vi "ERIO RT Send Notification Messages.vi"(8 "error in (no error)":errorcluster, 9 "AWS Variables In":T1, 10 "Message Body":string, 11 "Supervisory Variables In":T2={"Alarm Threshold"=0.0, "Shutdown"=FALSE, "Enable SNS Alarm"=FALSE, "Enable SNS Stage Notification"=FALSE, "Enable SQS Notification"=FALSE, "Enable S3 TDMS Signal Capture"=FALSE, "Enable SystemLink Signal Capture"=FALSE, "Capture Signal"=FALSE, "Server Update"=FALSE, "AWS Access Key"="", "AWS Secret Key"="", "Phone Number"="", "Region"=enum."us-east-1", "AWS SQS Queue"="mynicloud-demotest2", "AWS S3 Bucket"="mynicloud-demotest2"}) -> (0 "error out":errorcluster, 1 "AWS Variables Out":T1)   [LabVIEW 2017]
doc: "Send out relevant notification messages.\n\nJames Tillett PE\nEndeavor Engineering Inc.\nwww.endeavoreng.com"
uses:
  Controls/ERIO Supervisory Variables.ctl
  <vilib>/AWS Toolkit/Core/HTTP Request/Region.ctl
  Controls/ERIO AWS Toolkit Variables.ctl
  <vilib>/AWS Toolkit/SQS/Queue/Queue.lvclass
  <vilib>/AWS Toolkit/SNS/Phone Number/Phone Number.lvclass
  <vilib>/AWS Toolkit/S3/Bucket/Bucket.lvclass
  <vilib>/AWS Toolkit/Core/HTTP Request/HTTP Request.lvclass
panel:
  out "Supervisory Variables oUT":T2={"Alarm Threshold"=0.0, "Shutdown"=FALSE, "Enable SNS Alarm"=FALSE, "Enable SNS Stage Notification"=FALSE, "Enable SQS Notification"=FALSE, "Enable S3 TDMS Signal Capture"=FALSE, "Enable SystemLink Signal Capture"=FALSE, "Capture Signal"=FALSE, "Server Update"=FALSE, "AWS Access Key"="", "AWS Secret Key"="", "Phone Number"="", "Region"=enum."us-east-1", "AWS SQS Queue"="mynicloud-demotest2", "AWS S3 Bucket"="mynicloud-demotest2"}
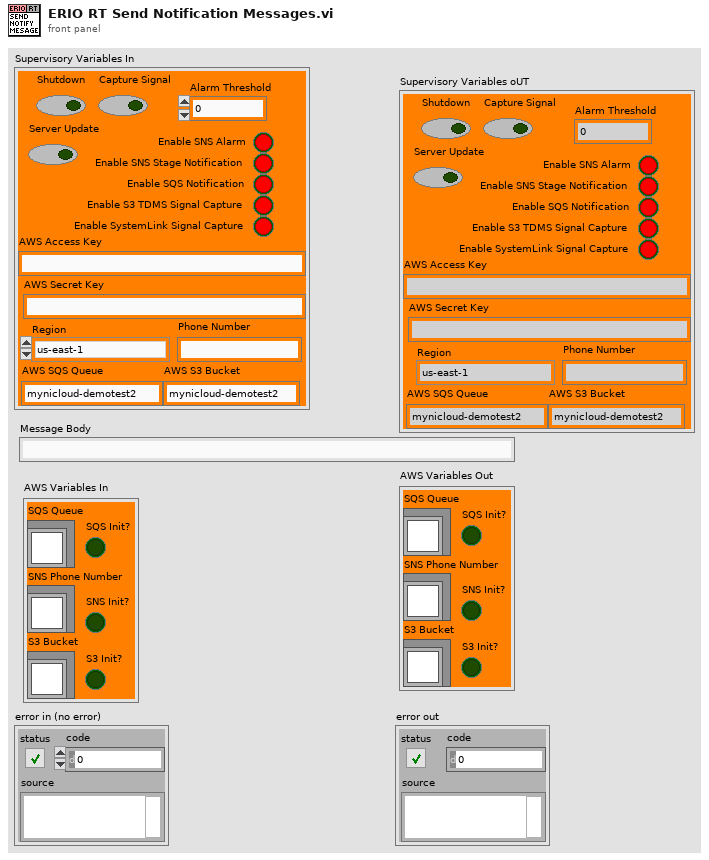
[diagram p1: front panel]
types:
  T1 = typedef "ERIO AWS Toolkit Variables.ctl" = cluster{"SQS Queue":refnum<class "Queue.lvclass">, "SNS Phone Number":refnum<class "Phone Number.lvclass">, "S3 Bucket":refnum<class "Bucket.lvclass">, "SQS Init?":bool, "S3 Init?":bool, "SNS Init?":bool}
  T2 = typedef "ERIO Supervisory Variables.ctl" = cluster{"Alarm Threshold":dbl, "Shutdown":bool, "Enable SNS Alarm":bool, "Enable SNS Stage Notification":bool, "Enable SQS Notification":bool, "Enable S3 TDMS Signal Capture":bool, "Enable SystemLink Signal Capture":bool, "Capture Signal":bool, "Server Update":bool, "AWS Access Key":string, "AWS Secret Key":string, "Phone Number":string, "Region":T3, "AWS SQS Queue":string, "AWS S3 Bucket":string}
  T3 = typedef "NI_AWS_Core.lvlib/HTTP Request.lvclass/Region.ctl" = enum16{"us-east-1", "us-east-2", "us-west-1", "us-west-2", "ap-northeast-1", "ap-northeast-2", "ap-southeast-1", "ap-southeast-2", "ca-central-1", "eu-central-1", "eu-west-1", "eu-west-2", "sa-east-1"}
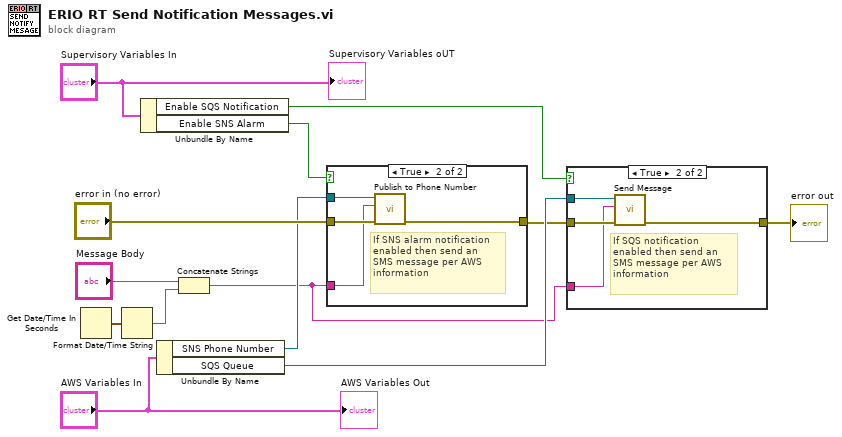
[diagram p0: block diagram]
diagram:
  n1 = Get Date/Time In Seconds() -> (seconds since 1Jan1904=w10:timestamp)
  n2 = Format Date/Time String(seconds (now)=w10) -> (date/time string=w11:string)  [unwired: 2 in]
  n3 = Unbundle By Name("Supervisory Variables In") -> ("Enable SQS Notification"=w7:bool, "Enable SNS Alarm"=w8:bool)
  n4 = Unbundle By Name("AWS Variables In") -> ("SNS Phone Number"=w12:refnum<class "Phone Number.lvclass">, "SQS Queue"=w6:refnum<class "Queue.lvclass">)
  n5 = Concatenate Strings("Message Body", w11) -> (w4:string)
  n6 = case shown="True" w8 {
    tunnel: "error in (no error)" -> [w14 w17]
    tunnel: [w14 w18] -> w5
    tunnel: w12 -> [_ w16]
    tunnel: w4 -> [_ w15]
    frame False {
    }
    frame True {
      # "If SNS alarm notification \nenabled then send an\nSMS message per AWS \ninformation"
      n7 = call <vilib>:"Publish to Phone Number.vi"("error in (no error)"=w17, "Message"=w15, "Phone Number in"=w16) -> ("error out"=w18:errorcluster)  [unwired: 7 in, 1 out]
    }
  }
  n8 = case shown="True" w7 {
    tunnel: w5 -> [w19 w22]
    tunnel: [w19 w23] -> w2
    tunnel: w6 -> [_ w21]
    tunnel: w4 -> [_ w20]
    frame False {
    }
    frame True {
      # "If SQS notification \nenabled then send an\nSMS message per AWS \ninformation"
      n9 = call <vilib>:"Send Message.vi"("error in (no error)"=w22, "Message Body"=w20, "SQS in"=w21) -> ("error out"=w23:errorcluster)  [unwired: 4 in, 4 out]
    }
  }
  "error out" <- w2
  "Supervisory Variables oUT" <- "Supervisory Variables In"
  "AWS Variables Out" <- "AWS Variables In"
